vi "Generate Holonomic Thetas.vi"(6 "WayPoints":T1, 8 "time unflat":cluster{dbl[]}[](array[cluster]), 9 "dt":dbl, 11 "Angular Limits":T2={"Velocity (deg/s)"=6.0, "Accel (deg/s^2)"=15.0, "Jerk (deg/s^3)"=150.0} {"Jerk (deg/s^3)" min=0.0 step=1.0; "Accel (deg/s^2)" min=0.0; "Velocity (deg/s)" min=0.0}) -> (2 "X":dbl[](array[numeric]), 3 "V":dbl[](array[numeric]))   [LabVIEW 2025]
uses:
  Types/Angluar Limits.ctl
  Types/Waypoints.ctl
panel:
  out "x*y 2":dbl
  out "x*y":dbl
  out "Waveform Chart 2":dbl[](graph)
  out "Waveform Chart":dbl[](graph)
  out "output variable":i32
  out "size(s) 2":i32
  out "size(s)":i32
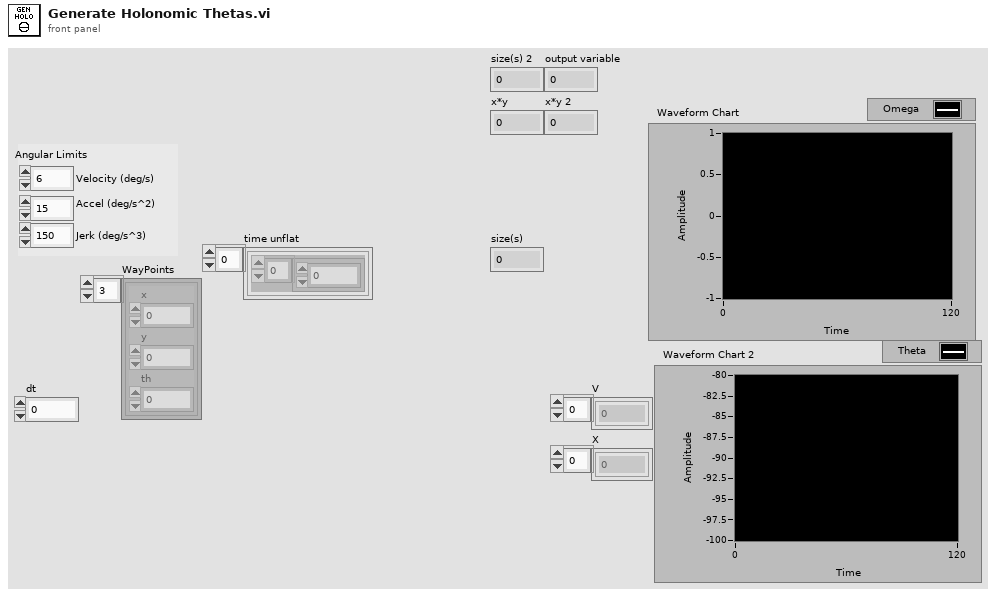
[diagram p1: front panel]
types:
  T1 = typedef "Waypoints.ctl" = cluster{"x":sgl, "y":sgl, "th":sgl}[]
  T2 = typedef "Angluar Limits.ctl" = cluster{"Velocity (deg/s)":dbl, "Accel (deg/s^2)":dbl, "Jerk (deg/s^3)":dbl}
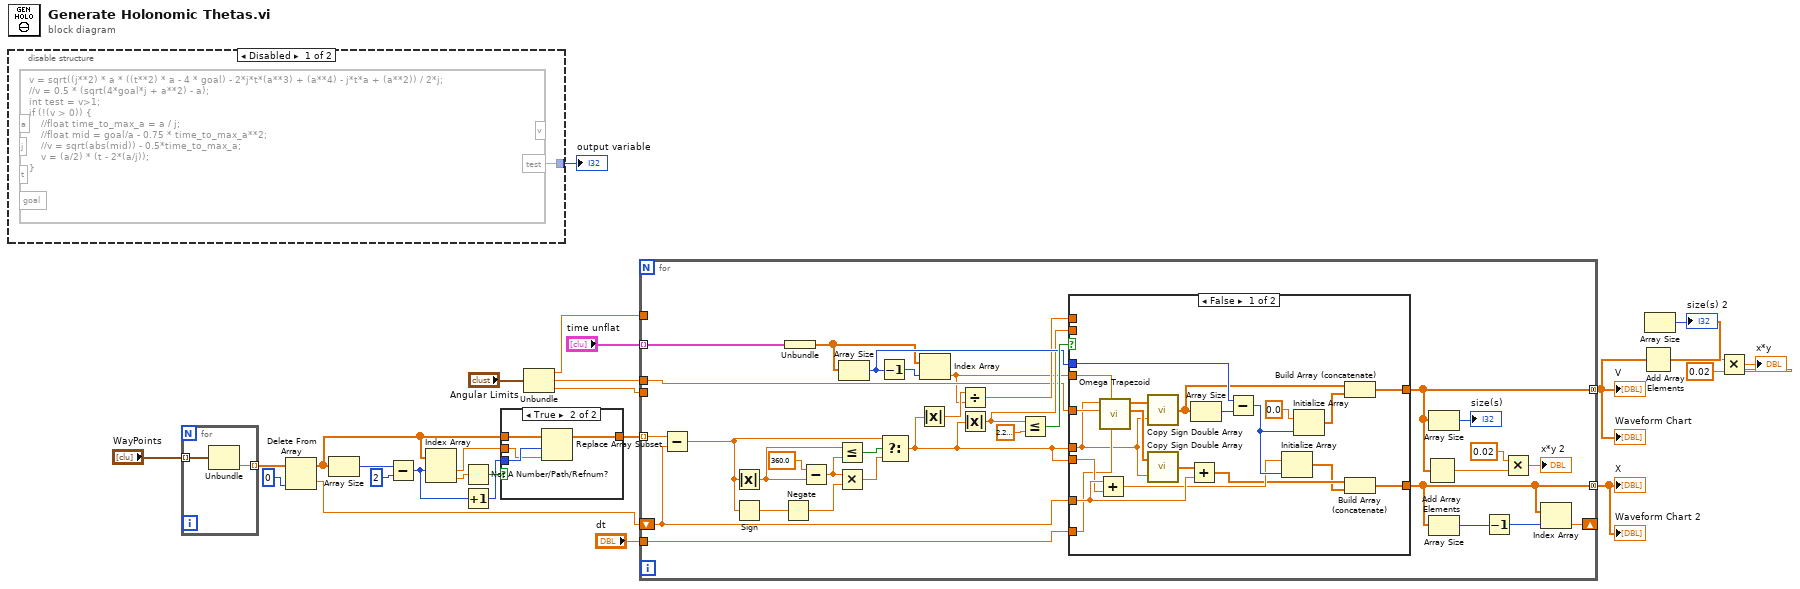
[diagram p0: block diagram]
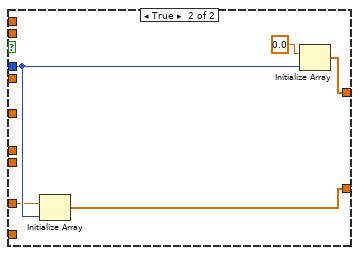
[diagram p4: hidden frame]
diagram:
  n1 = disable-structure shown="Disabled" {
    disable-tunnel: [w27 _] -> w19
    frame Disabled {
      n2 = formula code="v = sqrt((j**2) * a * ((t**2) * a - 4 * goal) - 2*j*t*(a**3) + (a**4) - j*t*a + (a**2)) / 2*j;\n//v = 0.5 * (sqrt(4*goal*j + a**2) - a);\nint test = v>1;\nif (!(v > 0)) {\n    //float time_to_max_a = a / j;\n    //float mid = goal/a - 0.75 * time_to_max_a**2;\n    //v = sqrt(abs(mid)) - 0.5*time_to_max_a;\n    v = (a/2) * (t - 2*(a/j));\n}"() -> ("test"=w27:i32)  [unwired: 4 in, 1 out]
    }
    frame Enabled {
    }
  }
  "output variable" <- w19
  n3 = for {
    tunnel: "WayPoints" -> [w29] mode=indexing
    tunnel: [w28] -> w18 mode=indexing
    n4 = Unbundle(w29) -> ("th"=w28:sgl)  [unwired: 2 out]
  }
  n5 = Delete From Array(array=w18, index=0) -> (deleted portion=w16:sgl, array with subset deleted=w14:sgl[])  [unwired: 1 in]
  n6 = Array Size(array=w14) -> (size(s)=w13:i32)
  n7 = Subtract(x=w13, y=2) -> (x-y=w10:i32)
  n8 = Index Array(array=w14, index #1=w10) -> (element #1=w8:sgl, element #2=w11:sgl)  [unwired: 1 in]
  n9 = Not A Number/Path/Refnum?(number/path/refnum=w11) -> (NaN/Path/Refnum?=w15:bool)
  n10 = Increment(x=w10) -> (x+1=w9:i32)
  n11 = case shown="True" w15 {
    tunnel: w14 -> [w30 w34]
    tunnel: w9 -> [_ w33]
    tunnel: w8 -> [_ w32]
    tunnel: [w30 w31] -> w7
    frame False {
    }
    frame True {
      n12 = Replace Array Subset(array=w34, new element=w32, index=w33) -> (w31:sgl[])
    }
  }
  n13 = Unbundle("Angular Limits") -> ("Velocity (deg/s)"=w26:dbl, "Accel (deg/s^2)"=w24:dbl, "Jerk (deg/s^3)"=w25:dbl)
  n14 = for {
    tunnel: w26 -> [_]
    tunnel: w25 -> [_]
    tunnel: w24 -> [w40]
    tunnel: w7 -> [w62] mode=indexing
    shift-right: [w54] -> _
    shift-left: w16 -> [w58]
    tunnel: "dt" -> [w52]
    tunnel: "time unflat" -> [w61] mode=indexing
    tunnel: [w38] -> w4 mode=concatenating
    tunnel: [w57] -> w5 mode=concatenating
    n15 = Subtract(x=w62, y=w58) -> (x-y=w45:dbl)
    n16 = Absolute Value(x=w45) -> (abs(x)=w47:dbl)
    n17 = Sign(1:w45) -> (0:w44:dbl)
    n18 = Negate(x=w44) -> (-x=w43:dbl)
    n19 = Unbundle(w61) -> (w60:dbl[])
    n20 = Subtract(x=360.0, y=w47) -> (x-y=w46:dbl)
    n21 = Less Or Equal?(x=w47, y=w46) -> (x <= y?=w48:bool)
    n22 = Multiply(x=w46, y=w43) -> (x*y=w42:dbl)
    n23 = Array Size(array=w60) -> (size(s)=w63:i32)
    n24 = Decrement(x=w63) -> (x-1=w64:i32)
    n25 = Select(t=w45, s=w48, f=w42) -> (s? t:f=w41:dbl)
    n26 = Absolute Value(x=w41) -> (abs(x)=w51:dbl)
    n27 = Index Array(array=w60, index=w64) -> (element=w39:dbl)
    n28 = Divide(x=w51, y=w39) -> (x/y=w50:dbl)
    n29 = Absolute Value(x=w41) -> (abs(x)=w53:dbl)
    n30 = Less Or Equal?(x=w53, y=2.220446049250313e-16) -> (x <= y?=w65:bool)
    n31 = case shown="False" w65 {
      tunnel: [w77 w91] -> w38
      tunnel: [w74 w89] -> w57
      tunnel: w63 -> [w85 w88]
      tunnel: w58 -> [w81 w87]
      tunnel: w41 -> [w68 _]
      tunnel: w41 -> [w73 _]
      tunnel: w53 -> [_ _]
      tunnel: w52 -> [w69 _]
      tunnel: w50 -> [_ _]
      tunnel: w40 -> [w70 _]
      tunnel: w39 -> [w67 _]
      frame False {
        n32 = Add(x=w81, y=w73) -> (x+y=w80:dbl)
        n33 = call "Omega Trapezoid.vi"("dt"=w69, "ttot"=w67, "a"=w70, "g"=w68) -> ("Thetas"=w71:dbl[], "Omegas"=w72:dbl[])  [unwired: 6 in]
        n34 = call "Copy Sign Double Array.vi"("y"=w68, "x"=w72) -> ("x out"=w79:dbl[])
        n35 = call "Copy Sign Double Array.vi"("y"=w68, "x"=w71) -> ("x out"=w86:dbl[])
        n36 = Add(x=w86, y=w81) -> (x+y=w76:dbl[])
        n37 = Array Size(array=w79) -> (size(s)=w84:i32)
        n38 = Subtract(x=w85, y=w84) -> (x-y=w83:i32)
        n39 = Initialize Array(w80, w83) -> (w75:dbl[])
        n40 = Initialize Array(0.0 ("element"), w83) -> (w78:dbl[])
        n41 = Build Array (concatenate)(w79, w78) -> (w77:dbl[])
        n42 = Build Array (concatenate)(w76, w75) -> (w74:dbl[])
      }
      frame True {
        n43 = Initialize Array(w87, w88) -> (w89:dbl[])
        n44 = Initialize Array(0.0 ("element"), w88) -> (w91:dbl[])
      }
    }
    n45 = Add Array Elements(numeric array=w38) -> (sum=w37:dbl)
    n46 = Array Size(array=w38) -> (size(s)=→"size(s)":i32)
    n47 = Array Size(array=w57) -> (size(s)=w56:i32)
    n48 = Decrement(x=w56) -> (x-1=w55:i32)
    n49 = Multiply(x=0.02 ("y"), y=w37) -> (x*y=→"x*y 2":dbl)
    n50 = Index Array(array=w57, index=w55) -> (element=w54:dbl)
  }
  "V" <- w4
  "X" <- w5
  "Waveform Chart" <- w4
  "Waveform Chart 2" <- w5
  n51 = Add Array Elements(numeric array=w4) -> (sum=w3:dbl)
  n52 = Array Size(array=w4) -> (size(s)=→"size(s) 2":i32)
  n53 = Multiply(x=w3, y=0.02) -> (x*y=→"x*y":dbl)
